vi "New ROI and Overlay Selection.vi"(8 "error in (no error)":errorcluster, 10 "ItemTag":string, 11 "IMAQ Display in":refnum<class "HIJ Vision Display.lvclass">) -> (0 "error out":errorcluster, 3 "IMAQ Display out":refnum<class "HIJ Vision Display.lvclass">)   [LabVIEW 2020, in "HIJ Vision Display.lvlib" / "HIJ Vision Display.lvclass"]
uses:
  HIJ Vision Display.lvclass
  HIJ Vision Display.lvclass/HIJ Vision Display.ctl
  <vilib>/ActorFramework/Actor/Actor.lvclass
  Application Base Actors/HIJ Vision Application/HIJ Vision Application Messages/Set Result Settings Msg/Set Result Settings Msg.lvclass
  C:/Users/AlexK/work/LabVIEW Programme/POLARIS-AS-3-Cams/Submodules/Viewable Actor/ViewableActor/ViewableActor.lvclass
  C:/Program Files (x86)/National Instruments/LabVIEW 2020/vi.lib/ActorFramework/Actor/Actor.lvclass
  C:/Users/AlexK/work/LabVIEW Programme/POLARIS-AS-3-Cams/Submodules/HIJ Vision/Display Actors/HIJ Vision Display/HIJ Vision Display/HIJ Vision Display.lvclass
  C:/Users/AlexK/work/LabVIEW Programme/POLARIS-AS-3-Cams/Submodules/HIJ Vision/Analyze/Analyze Actor/IAnalysis/IAnalysis.lvclass
  C:/Users/AlexK/work/LabVIEW Programme/POLARIS-AS-3-Cams/Submodules/HIJ Vision/Camera Actors/Camera Actor/ICamera/ICamera.lvclass
  Analyze/Results and Overlays/Results Base/Analyze Results Base.lvclass
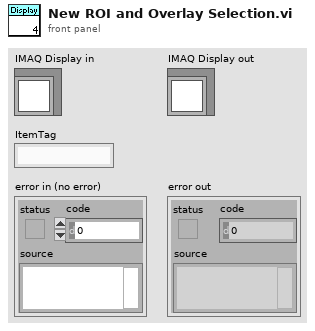
[diagram p1: front panel]
types:
  T1 = typedef "HIJ Vision Display.lvlib/HIJ Vision Display.lvclass/Named ROI.ctl" = cluster{"ROI":cluster{"Global Rectangle":i32[], "Contours":cluster{"Contour Type":u32, "ROI Type":u32, "Points":i32[]}[]}, "Name":string}
  T2 = cluster{"Global Rectangle":i32[], "Contours":cluster{"Contour Type":u32, "ROI Type":u32, "Points":i32[]}[]}
  T3 = typedef "IMAQ Image.ctl" = refnum<image>
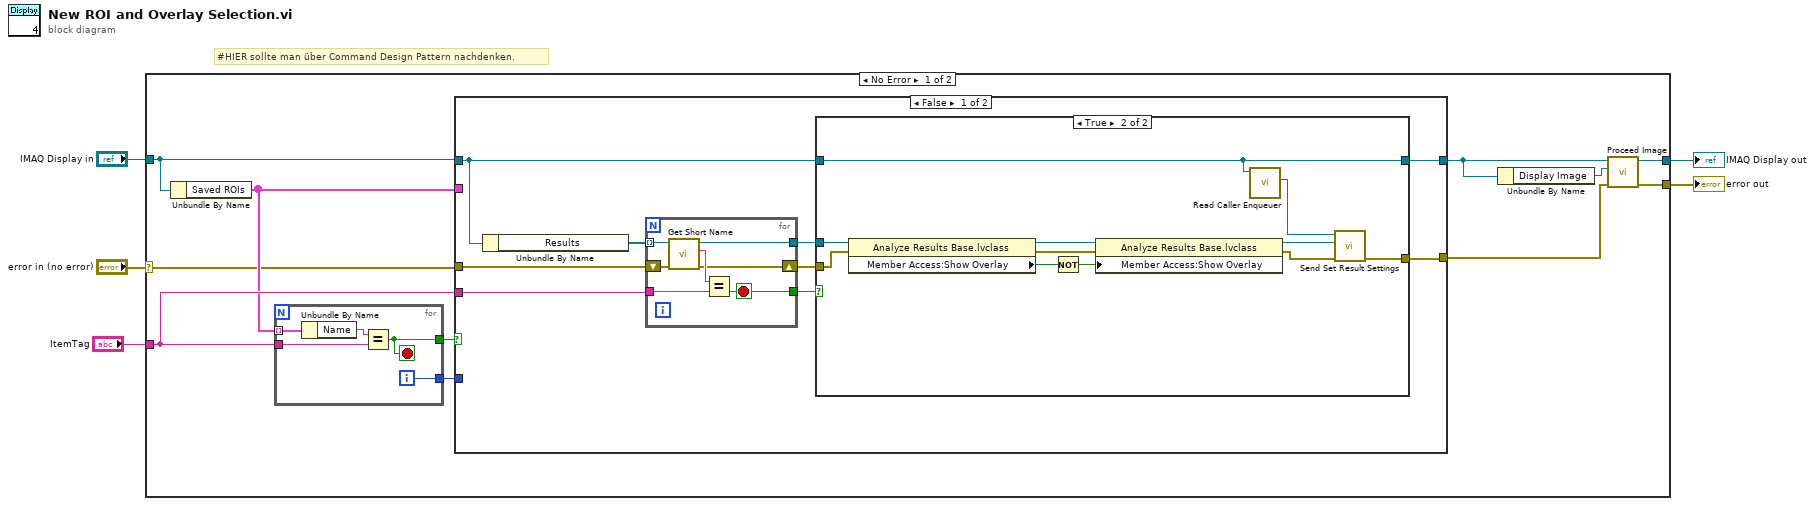
[diagram p0: block diagram]
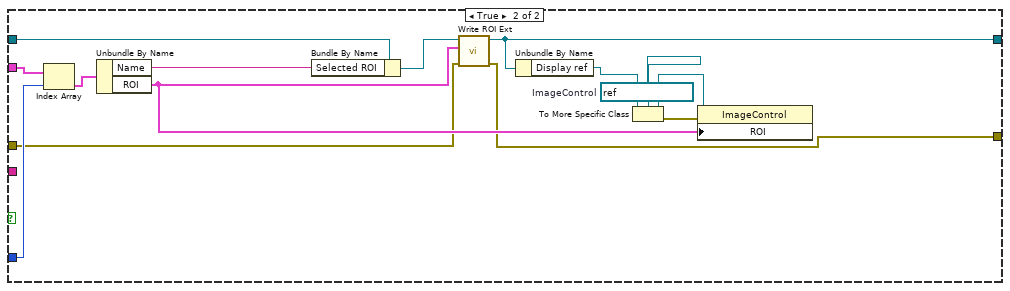
[diagram p3: hidden frame]
diagram:
  # "#HIER sollte man über Command Design Pattern nachdenken."
  n1 = case shown="No Error" "error in (no error)" {
    selector: "error in (no error)" -> [w7 w66]
    tunnel: [w8 w66] -> w4
    tunnel: [w11 w65] -> w1
    tunnel: "IMAQ Display in" -> [w12 w65]
    tunnel: "ItemTag" -> [w16 _]
    frame No Error {
      n2 = Unbundle By Name(w12) -> ("Saved ROIs"=w15:T1[])
      n3 = for {
        tunnel: w15 -> [w64] mode=indexing
        tunnel: w16 -> [w62]
        tunnel: [w61] -> w13
        tunnel: [w60] -> w14
        i -> [w60]
        stop <- w61 stop-if-true
        n4 = Unbundle By Name(w64) -> ("Name"=w63:string)
        n5 = Equal?(x=w63, y=w62) -> (x = y?=w61:bool)
      }
      n6 = case shown="False" w13 {
        tunnel: w15 -> [_ w58]
        tunnel: w14 -> [_ w59]
        tunnel: w12 -> [w25 w56]
        tunnel: w16 -> [w21 _]
        tunnel: [w24 w49] -> w10
        tunnel: w7 -> [w18 w47]
        tunnel: [w23 w46] -> w6
        frame False {
          n7 = Unbundle By Name(w25) -> ("Results"=w22:refnum<class "Analyze Results Base.lvclass">[])
          n8 = for {
            tunnel: w22 -> [w32] mode=indexing
            tunnel: w21 -> [w30]
            tunnel: [w29] -> w20
            tunnel: [w28] -> w19
            shift-right: [w26] -> w17
            shift-left: w18 -> [w27]
            stop <- w29 stop-if-true
            n9 = call-dynamic "Get Short Name.vi"("error in (no error)"=w27, "Analyze Results Base in"=w32) -> ("error out"=w26:errorcluster, "Short Name"=w31:string, "Analyze Results Base out"=w28:refnum<class "Analyze Results Base.lvclass">)  [unwired: 7 in]
            n10 = Equal?(x=w31, y=w30) -> (x = y?=w29:bool)
          }
          n11 = case shown="True" w20 {
            tunnel: w19 -> [_ w42]
            tunnel: w17 -> [w33 w40]
            tunnel: w25 -> [w34 w39]
            tunnel: [w34 w39] -> w24
            tunnel: [w33 w37] -> w23
            frame False {
            }
            frame True {
              n12 = property class="Analyze Results Base.lvclass"(reference=w42, error in=w40) -> (reference out=w45:refnum<class "Analyze Results Base.lvclass">, error out=w41:errorcluster, "Member Access:Show Overlay"=w44:bool)
              n13 = Not(x=w44) -> (.not. x?=w43:bool)
              n14 = property class="Analyze Results Base.lvclass"(reference=w45, error in=w41, "Member Access:Show Overlay"=w43) -> (reference out=w36:refnum<class "Analyze Results Base.lvclass">, error out=w35:errorcluster)
              n15 = call <vilib>:"Read Caller Enqueuer.vi"("Actor"=w39) -> ("Caller Enqueuer"=w38:refnum<class "Message Enqueuer.lvclass">)  [unwired: 10 in]
              n16 = call "Send Set Result Settings.vi"("error in (no error)"=w35, "Analyze Results"=w36, "Message Enqueuer"=w38) -> ("error out"=w37:errorcluster)  [unwired: 7 in, 1 out]
            }
          }
        }
        frame True {
          w51 = refnum<vi> refnum  # ImageControl
          n17 = Index Array(array=w58, index=w59) -> (element=w57:T1)
          n18 = Unbundle By Name(w57) -> ("Name"=w55:string, "ROI"=w48:T2)
          n19 = Bundle By Name(cluster=w56, "Selected ROI"=w55) -> (w54:refnum<class "HIJ Vision Display.lvclass">)
          n20 = call "Write ROI Ext.vi"("error in (no error)"=w47, "ROI Descriptor"=w48, "IMAQ Display in"=w54) -> ("error out"=w46:errorcluster, "IMAQ Display out"=w49:refnum<class "HIJ Vision Display.lvclass">)  [unwired: 7 in]
          n21 = Unbundle By Name(w49) -> ("Display ref"=w53:refnum<vi>)
          n22 = To More Specific Class(target class=w51, reference=w53) -> (specific class reference=w52:refnum<vi>, error out=w50:errorcluster)  [unwired: 1 in]
          n23 = property class="ImageControl"(reference=w52, error in=w50, "ROI"=w48) -> ()  [unwired: 2 out]
        }
      }
      n24 = Unbundle By Name(w10) -> ("Display Image"=w9:T3)
      n25 = call "Proceed Image.vi"("error in (no error)"=w6, "Image"=w9, "IMAQ Display in"=w10) -> ("error out"=w8:errorcluster, "HIJ Vision Display out"=w11:refnum<class "HIJ Vision Display.lvclass">)  [unwired: 7 in]
    }
    frame Error {
    }
  }
  "error out" <- w4
  "IMAQ Display out" <- w1
